vi "pp2_loadTrial.vi"(0 "State In":T8={"Curr  tr"=0, "Curr (ms)"=0, "Cum (ms)"=0, "Run loop diff"=0, "Tone countdown (ms)"=0, "Countdown (ms)"=0, "Curr type"=0, "Curr State"=enum."0 Habituation", "Prev State"=enum."0 Habituation", "Null"=FALSE, "Sw1"=FALSE, "Tone\nGate"=FALSE, "Sw2"=FALSE, "Stim"=FALSE, "Current DAQ DO Int"=0, "Current Loaded Trial"={"Trial Type Number"=1, "Trial Type"=enum."GO", "Trial Weight"=100, "Shock (mA)"=0.3, "Duration (ms)"=0.25, "Type"=enum."04 FM Sweep", "Stim P2"=4000.0, "Stim P3"=0.0, "Stim P4"=0.0, "Stim P1"=2000.0}, "Next Trial"={"Trial Type Number"=1, "Trial Type"=enum."GO", "Trial Weight"=100, "Shock (mA)"=0.3, "Duration (ms)"=0.25, "Type"=enum."04 FM Sweep", "Stim P2"=4000.0, "Stim P3"=0.0, "Stim P4"=0.0, "Stim P1"=2000.0}} {"Current DAQ DO Int" format="%b"; "Next Trial"."Shock (mA)" min=-1.0 max=5.0; "Next Trial"."Trial Weight" step=1; "Next Trial"."Duration (ms)" min=0.0 max=1.0; "Next Trial"."Trial Type Number" min=1 max=256 step=1; "Current Loaded Trial"."Shock (mA)" min=-1.0 max=5.0; "Current Loaded Trial"."Trial Weight" step=1; "Current Loaded Trial"."Duration (ms)" min=0.0 max=1.0; "Current Loaded Trial"."Trial Type Number" min=1 max=256 step=1; "Curr type" format="%#.6f"}, 1 "Session param (dynamic)":T7={"Def M shock (mA)"=400.0, "Def F shock (mA)"=0.0, "Def M shock +/-"=4, "Def F shock +/-"=4} {"Def F shock +/-" min=0 step=1; "Def M shock +/-" min=0 step=1}, 2 "Session List (Hidden variable)":u8[](array[numeric]), 3 "Trial Types":T1[](array[typedef])=[{"Trial Type Number"=1, "Trial Type"=enum."GO", "Trial Weight"=1, "Shock (mA)"=-1.0, "Duration (ms)"=250.0, "Type"=enum."04 FM Sweep", "Stim P2"=4000.0, "Stim P3"=0.0, "Stim P4"=0.0, "Stim P1"=2000.0}, {"Trial Type Number"=2, "Trial Type"=enum."NOGO", "Trial Weight"=1, "Shock (mA)"=-1.0, "Duration (ms)"=250.0, "Type"=enum."04 FM Sweep", "Stim P2"=2000.0, "Stim P3"=0.0, "Stim P4"=0.0, "Stim P1"=4000.0}] {"Shock (mA)" min=-1.0 max=5.0; "Trial Weight" step=1; "Duration (ms)" min=0.0 max=1.0; "Trial Type Number" min=1 max=256 step=1}, 5 "Daq config In":T4={"Sound AO"="Dev2/ao0", "Shock intesity AO"="Dev1/ao1", "Code/LED DO"="Dev1/port1:2", "Switches DI"="Dev1/port0/line0:1", "Webcam"="cam0", "Sound AO task"="", "Sound card task"=0, "Shock intensity AO task"="", "Code/LED DO task"="", "Switch DI task"="", "AO <=> Sound card"=FALSE, "Sound card"=0, "sample rate"=8000.0, "Variable shock"=FALSE, "Webcam on"=FALSE, "Tone gate PFI"="/Dev1/PFI1"} {"sample rate" min=8000.0; "Sound card task" format="%.0x"}, 11 "error in (no error)":errorcluster) -> (4 "State Out":T8={"Curr  tr"=0, "Curr (ms)"=0, "Cum (ms)"=0, "Run loop diff"=0, "Tone countdown (ms)"=0, "Countdown (ms)"=0, "Curr type"=0, "Curr State"=enum."0 Habituation", "Prev State"=enum."0 Habituation", "Null"=FALSE, "Sw1"=FALSE, "Tone\nGate"=FALSE, "Sw2"=FALSE, "Stim"=FALSE, "Current DAQ DO Int"=0, "Current Loaded Trial"={"Trial Type Number"=1, "Trial Type"=enum."GO", "Trial Weight"=100, "Shock (mA)"=0.3, "Duration (ms)"=0.25, "Type"=enum."04 FM Sweep", "Stim P2"=4000.0, "Stim P3"=0.0, "Stim P4"=0.0, "Stim P1"=2000.0}, "Next Trial"={"Trial Type Number"=1, "Trial Type"=enum."GO", "Trial Weight"=100, "Shock (mA)"=0.3, "Duration (ms)"=0.25, "Type"=enum."04 FM Sweep", "Stim P2"=4000.0, "Stim P3"=0.0, "Stim P4"=0.0, "Stim P1"=2000.0}} {"Current DAQ DO Int" format="%b"; "Next Trial"."Shock (mA)" min=-1.0 max=5.0; "Next Trial"."Trial Weight" step=1; "Next Trial"."Duration (ms)" min=0.0 max=1.0; "Next Trial"."Trial Type Number" min=1 max=256 step=1; "Current Loaded Trial"."Shock (mA)" min=-1.0 max=5.0; "Current Loaded Trial"."Trial Weight" step=1; "Current Loaded Trial"."Duration (ms)" min=0.0 max=1.0; "Current Loaded Trial"."Trial Type Number" min=1 max=256 step=1; "Curr type" format="%#.6f"}, 6 "Daq config Out":T4={"Sound AO"="Dev2/ao0", "Shock intesity AO"="Dev1/ao1", "Code/LED DO"="Dev1/port1:2", "Switches DI"="Dev1/port0/line0:1", "Webcam"="cam0", "Sound AO task"="", "Sound card task"=0, "Shock intensity AO task"="", "Code/LED DO task"="", "Switch DI task"="", "AO <=> Sound card"=FALSE, "Sound card"=0, "sample rate"=8000.0, "Variable shock"=FALSE, "Webcam on"=FALSE, "Tone gate PFI"="/Dev1/PFI1"} {"sample rate" min=8000.0; "Sound card task" format="%.0x"}, 15 "error out":errorcluster)   [LabVIEW 2013]
uses:
  <vilib>/DAQmx/configure/trigger.llb/DAQmx Start Trigger (Digital Edge).vi
  <vilib>/DAQmx/write.llb/DAQmx Write (Analog Wfm 1Chan NSamp).vi
  <vilib>/DAQmx/configure/timing.llb/DAQmx Timing (Sample Clock).vi
  <vilib>/DAQmx/write.llb/DAQmx Write (Analog DBL 1Chan 1Samp).vi
  pp2_CTL_State.ctl
  pp2_CTL_StateInfo.ctl
  pp2_TrialType.ctl
  labolabo2/waveforms/WFTypes.ctl
  pp2_Trial.ctl
  pp2_CTL_SessionParamDynamic.ctl
  <vilib>/sound2/lvsound2.llb/Sound Output Task ID.ctl
  <vilib>/userdefined/High Color/IMAQdx.ctl
  pp2_CTL_DaqConfig.ctl
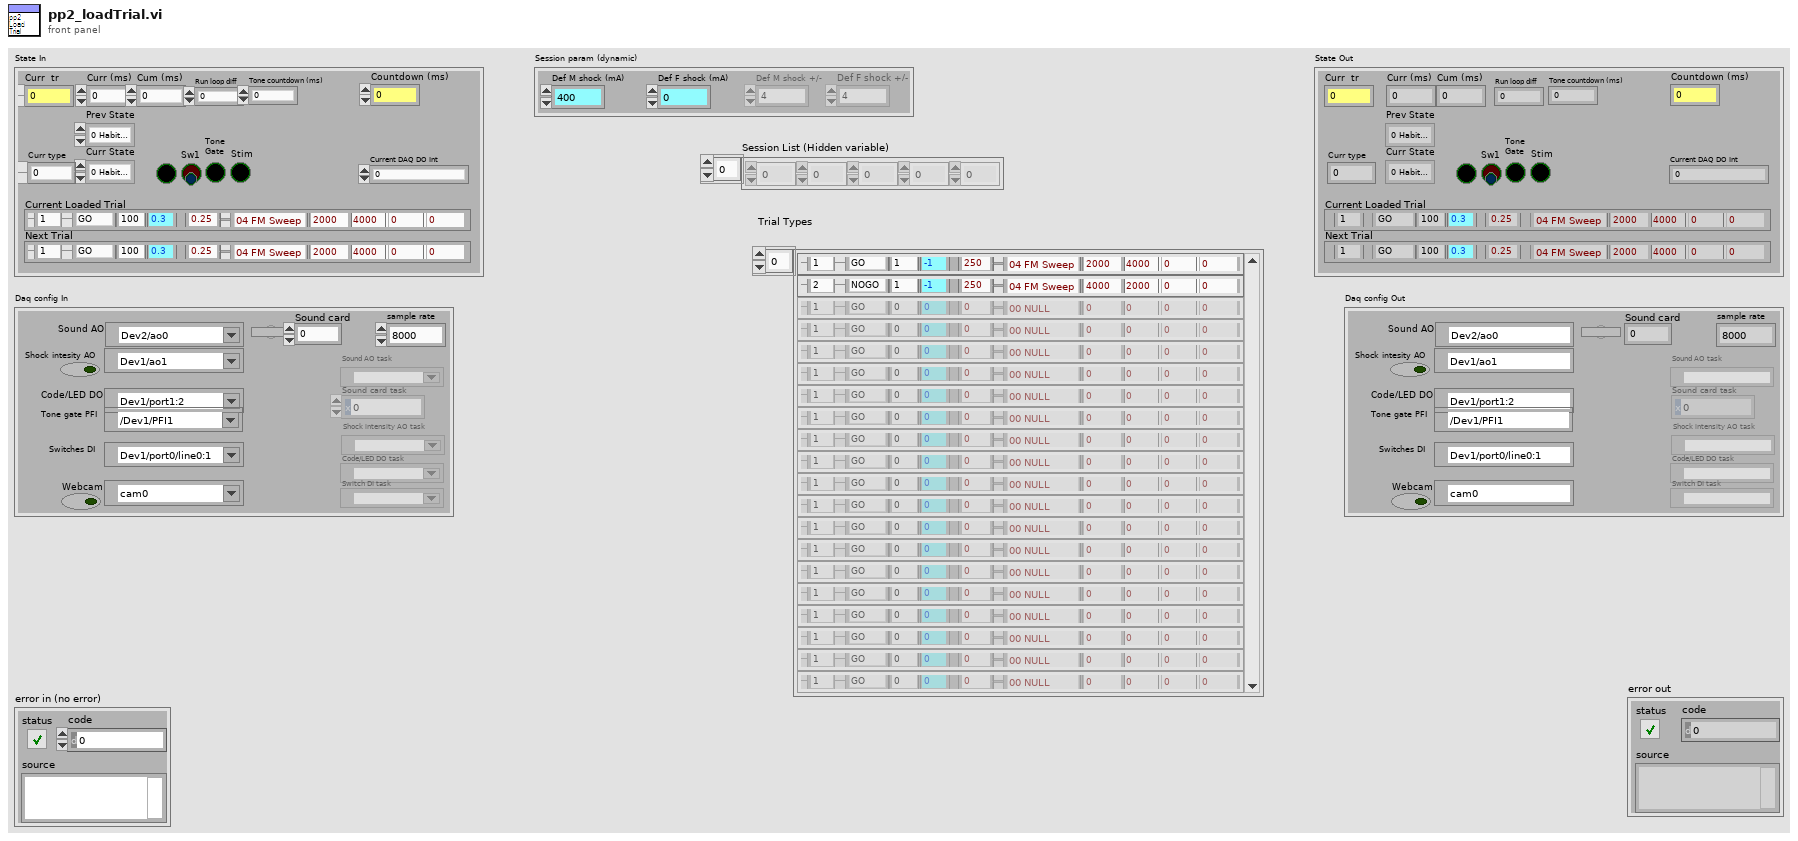
[diagram p1: front panel]
types:
  T1 = typedef "pp2_Trial.ctl" = cluster{"Trial Type Number":i16, "Trial Type":T2, "Trial Weight":u32, "Shock (mA)":dbl, "Duration (ms)":dbl, "Type":T3, "Stim P2":dbl, "Stim P3":dbl, "Stim P4":dbl, "Stim P1":dbl}
  T2 = typedef "pp2_TrialType.ctl" = enum16{"OFF", "GO", "NOGO", "TEST"}
  T3 = typedef "WFTypes.ctl" = enum16{"00 NULL", "01 DC", "02 Noise", "03 Pure Tone", "04 FM Sweep"}
  T4 = typedef "pp2_CTL_DaqConfig.ctl" = cluster{"Sound AO":tag, "Shock intesity AO":tag, "Code/LED DO":tag, "Switches DI":tag, "Webcam":T5, "Sound AO task":refnum<k21>, "Sound card task":T6, "Shock intensity AO task":refnum<k21>, "Code/LED DO task":refnum<k21>, "Switch DI task":refnum<k21>, "AO <=> Sound card":bool, "Sound card":u32, "sample rate":dbl, "Variable shock":bool, "Webcam on":bool, "Tone gate PFI":tag}
  T5 = typedef "IMAQdx.ctl" = refnum<k21>
  T6 = typedef "Sound Output Task ID.ctl" = u32
  T7 = typedef "pp2_CTL_SessionParamDynamic.ctl" = cluster{"Def M shock (mA)":dbl, "Def F shock (mA)":dbl, "Def M shock +/-":i32, "Def F shock +/-":i32}
  T8 = typedef "pp2_CTL_StateInfo.ctl" = cluster{"Curr  tr":u16, "Curr (ms)":i64, "Cum (ms)":i64, "Run loop diff":i64, "Tone countdown (ms)":i64, "Countdown (ms)":i64, "Curr type":u8, "Curr State":T9, "Prev State":T9, "Null":bool, "Sw1":bool, "Tone\nGate":bool, "Sw2":bool, "Stim":bool, "Current DAQ DO Int":u16, "Current Loaded Trial":T1, "Next Trial":T1}
  T9 = typedef "pp2_CTL_State.ctl" = enum8{"0 Habituation", "1 Load Trial", "2 Stay period", "3 Pre", "4 GO Trial", "5 GO Jumped", "6 GO Timeout", "7 NOGO Trial", "8 NOGO Jumped", "9 NOGO Timeout", "10 TEST Trial", "11 TEST Jumped", "12 TEST Timeout", "13 Intertrial Interval", "14 Done"}
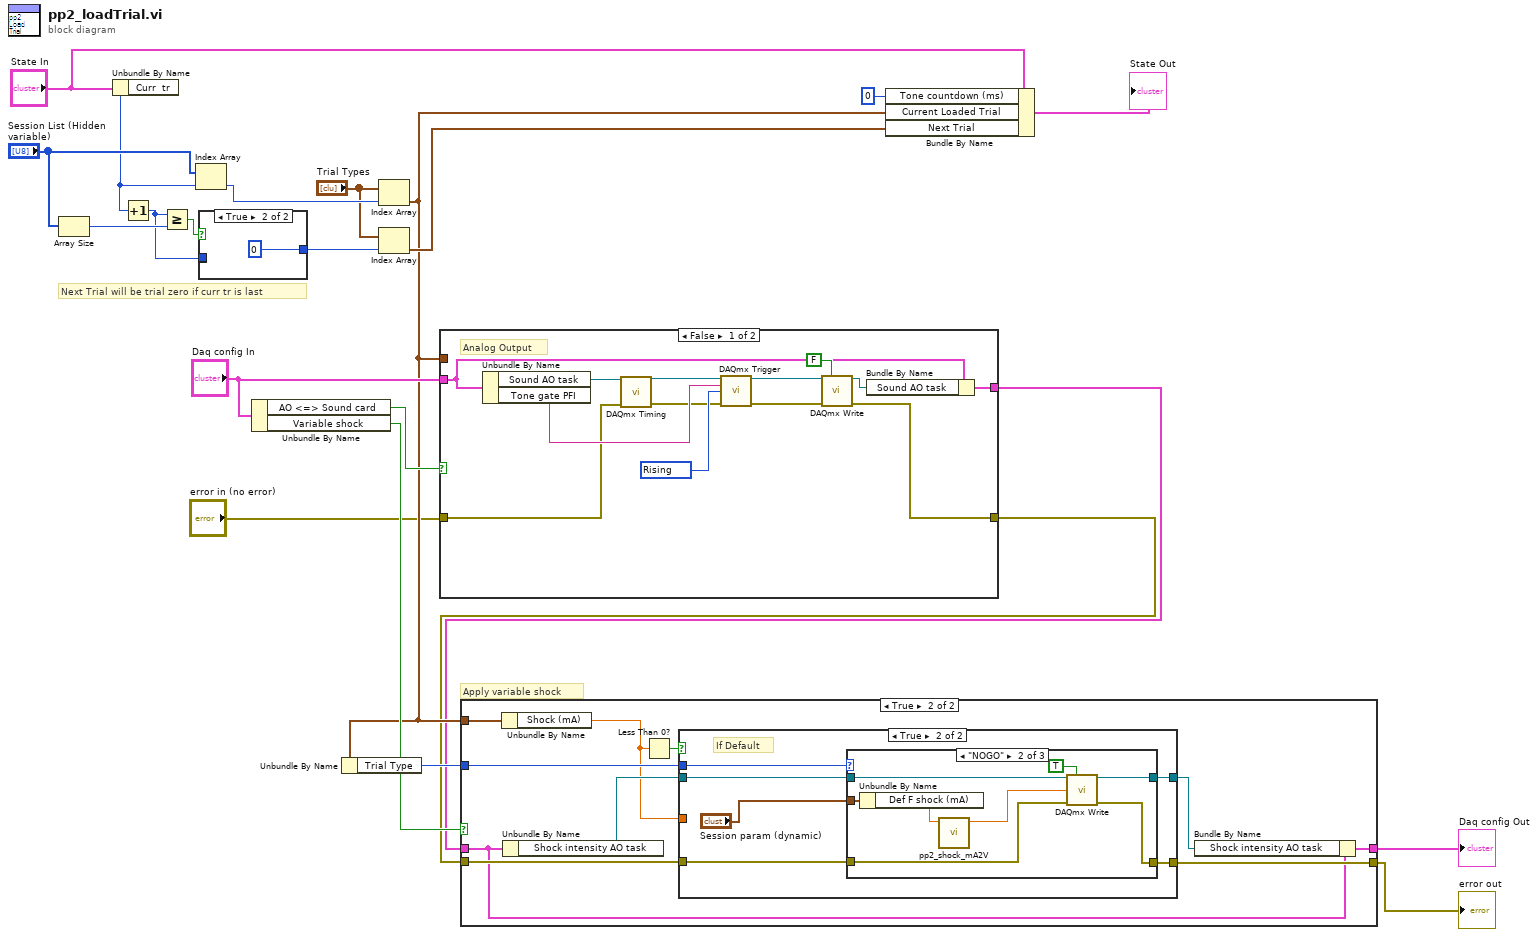
[diagram p0: block diagram]
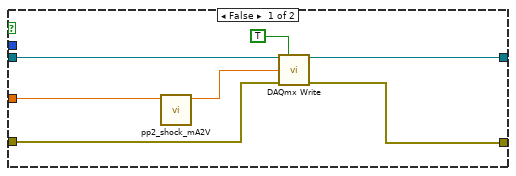
[diagram p3: hidden frame]
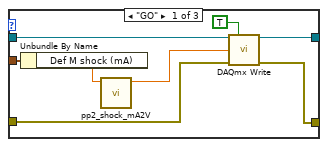
[diagram p4: hidden frame]
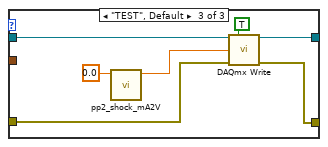
[diagram p5: hidden frame]
diagram:
  # "Next Trial will be trial zero if curr tr is last"
  # "Apply variable shock"
  n1 = Array Size(array="Session List (Hidden variable)") -> (size(s)=w16:i32)
  n2 = Unbundle By Name("State In") -> ("Curr  tr"=w14:u16)
  n3 = Increment(x=w14) -> (x+1=w13:u16)
  n4 = Greater Or Equal?(x=w13, y=w16) -> (x >= y?=w15:bool)
  n5 = Index Array(array="Session List (Hidden variable)", index=w14) -> (element=w18:u8)
  n6 = case shown="True" w15 {
    tunnel: w13 -> [w23 w25]
    tunnel: [_ w25] -> _
    tunnel: [w23 u8 0] -> w11
    frame False {
    }
    frame True {
    }
  }
  n7 = Unbundle By Name("Daq config In") -> ("AO <=> Sound card"=w20:bool, "Variable shock"=w19:bool)
  n8 = Index Array(array="Trial Types", index=w18) -> (element=w6:T1)
  n9 = Unbundle By Name(w6) -> ("Trial Type"=w7:T2)
  n10 = Index Array(array="Trial Types", index=w11) -> (element=w10:T1)
  n11 = case shown="False" w20 {
    tunnel: "Daq config In" -> [w30 _]
    tunnel: w6 -> [_ _]
    tunnel: [w29 _] -> w5
    tunnel: "error in (no error)" -> [w27 _]
    tunnel: [w26 _] -> w3
    frame False {
      w37 = 10280 items=["Rising"=10280, "Falling"=10171] ("edge")
      # "Analog Output"
      n12 = Unbundle By Name(w30) -> ("Sound AO task"=w31:refnum<k21>, "Tone gate PFI"=w38:tag)
      n13 = call-poly <vilib>:"DAQmx Timing.vi"("task/channels in"=w31, "error in"=w27) -> ("task out"=w35:refnum<k21>, "error out"=w36:errorcluster)  [unwired: 12 in]
      n14 = call-poly <vilib>:"DAQmx Trigger.vi"("task/channels in"=w35, "source"=w38, "edge"=w37, "error in"=w36) -> ("task out"=w34:refnum<k21>, "error out"=w33:errorcluster)  [unwired: 10 in]
      n15 = call-poly <vilib>:"DAQmx Write.vi"("task/channels in"=w34, "auto start"=FALSE, "error in"=w33) -> ("task out"=w28:refnum<k21>, "error out"=w26:errorcluster)  [unwired: 10 in, 1 out]
      n16 = Bundle By Name(cluster=w30, "Sound AO task"=w28) -> (w29:T4)
    }
    frame True {
    }
  }
  n17 = case shown="True" w19 {
    tunnel: w5 -> [w40 w45]
    tunnel: w6 -> [_ w50]
    tunnel: w3 -> [w39 w47]
    tunnel: [w39 w48] -> w1
    tunnel: w7 -> [_ w46]
    tunnel: [w40 w44] -> w2
    frame False {
    }
    frame True {
      n18 = Unbundle By Name(w50) -> ("Shock (mA)"=w41:dbl)
      n19 = Unbundle By Name(w45) -> ("Shock intensity AO task"=w49:refnum<k21>)
      n20 = Less Than 0?(x=w41) -> (x < 0?=w42:bool)
      n21 = case shown="True" w42 {
        tunnel: w46 -> [_ w63]
        tunnel: w49 -> [w56 w62]
        tunnel: [w51 w60] -> w48
        tunnel: w47 -> [w52 w59]
        tunnel: [w55 w58] -> w43
        tunnel: w41 -> [w53 _]
        frame False {
          n22 = call "pp2_shock_mA2V.vi"("Shock (mA)"=w53) -> ("Shock (V)"=w57:dbl)  [unwired: 10 in]
          n23 = call-poly <vilib>:"DAQmx Write.vi"("task/channels in"=w56, "auto start"=TRUE, "data"=w57, "error in"=w52) -> ("task out"=w55:refnum<k21>, "error out"=w51:errorcluster)  [unwired: 9 in, 1 out]
        }
        frame True {
          # "If Default"
          n24 = case shown="\"NOGO\"" w63 {
            tunnel: w62 -> [w71 w79 w86]
            tunnel: "Session param (dynamic)" -> [w70 w78 _]
            tunnel: [w67 w75 w84] -> w60
            tunnel: w59 -> [w66 w74 w83]
            tunnel: [w64 w73 w82] -> w58
            frame "GO" {
              n25 = Unbundle By Name(w70) -> ("Def M shock (mA)"=w69:dbl)
              n26 = call "pp2_shock_mA2V.vi"("Shock (mA)"=w69) -> ("Shock (V)"=w68:dbl)  [unwired: 10 in]
              n27 = call-poly <vilib>:"DAQmx Write.vi"("task/channels in"=w71, "auto start"=TRUE, "data"=w68, "error in"=w66) -> ("task out"=w64:refnum<k21>, "error out"=w67:errorcluster)  [unwired: 9 in, 1 out]
            }
            frame "NOGO" {
              n28 = Unbundle By Name(w78) -> ("Def F shock (mA)"=w77:dbl)
              n29 = call "pp2_shock_mA2V.vi"("Shock (mA)"=w77) -> ("Shock (V)"=w76:dbl)  [unwired: 10 in]
              n30 = call-poly <vilib>:"DAQmx Write.vi"("task/channels in"=w79, "auto start"=TRUE, "data"=w76, "error in"=w74) -> ("task out"=w73:refnum<k21>, "error out"=w75:errorcluster)  [unwired: 9 in, 1 out]
            }
            frame "TEST", Default {
              n31 = call "pp2_shock_mA2V.vi"("Shock (mA)"=0.0) -> ("Shock (V)"=w85:dbl)  [unwired: 10 in]
              n32 = call-poly <vilib>:"DAQmx Write.vi"("task/channels in"=w86, "auto start"=TRUE, "data"=w85, "error in"=w83) -> ("task out"=w82:refnum<k21>, "error out"=w84:errorcluster)  [unwired: 9 in, 1 out]
            }
          }
        }
      }
      n33 = Bundle By Name(cluster=w45, "Shock intensity AO task"=w43) -> (w44:T4)
    }
  }
  "Daq config Out" <- w2
  "error out" <- w1
  n34 = Bundle By Name(cluster="State In", "Tone countdown (ms)"=i64 0, "Current Loaded Trial"=w6, "Next Trial"=w10) -> (→"State Out":T8)
